vi "run.get.path.vi"(8 "error in":errorcluster, 11 "Run RID":string) -> (0 "error out":errorcluster, 3 "pah":string)   [LabVIEW 2020, in "Nominal Client.lvclass"]
uses:
  Nominal Client.lvclass
  Nominal Client.lvclass/Nominal Client.ctl
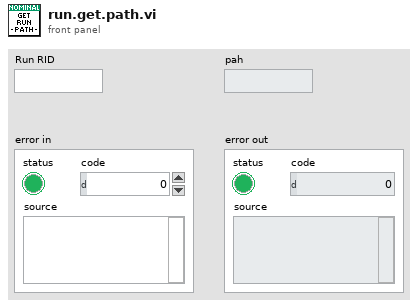
[diagram p1: front panel]
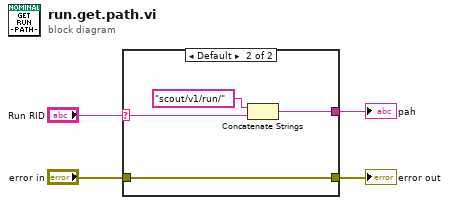
[diagram p0: block diagram]
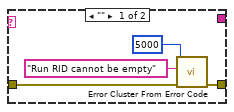
[diagram p2: hidden frame]
diagram:
  n1 = case shown="Default" "Run RID" {
    selector: "Run RID" -> [_ w11]
    tunnel: [_ w10] -> w1
    tunnel: "error in" -> [w8 w9]
    tunnel: [w6 w9] -> w2
    frame "" {
      n2 = call <vilib>:"Error Cluster From Error Code.vi"("error in (no error)"=w8, "error message (\"\")"="Run RID cannot be empty" ("error message (\"\")"), "error code (0)"=5000) -> ("error out"=w6:errorcluster)  [unwired: 6 in]
    }
    frame Default {
      n3 = Concatenate Strings("scout/v1/run/" ("path"), w11) -> (w10:string)
    }
  }
  "pah" <- w1
  "error out" <- w2
